vi "LoadProjectSettings.vi"(10 "SeqPath":string, 11 "Sequence Context In":refnum<k7>) -> (0 "error out":errorcluster, 2 "ProjectSettings":T1, 3 "Report Text":string)   [LabVIEW 2018]
uses:
  <vilib>/Utility/config.llb/Read Key (String).vi
  <vilib>/Utility/config.llb/Read Key (U32).vi
  <vilib>/Utility/config.llb/NI_LVConfig.lvlib
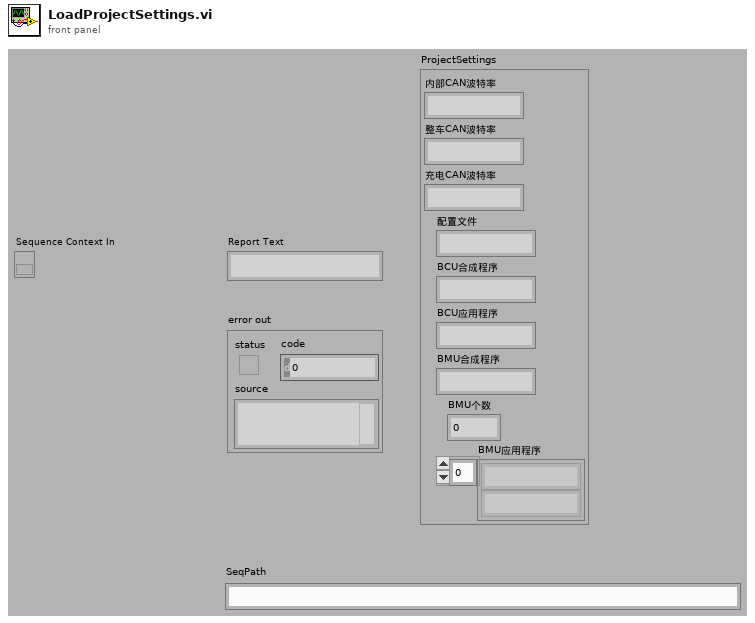
[diagram p1: front panel]
types:
  T1 = cluster{"内部CAN波特率":string, "整车CAN波特率":string, "充电CAN波特率":string, "配置文件":string, "BCU合成程序":string, "BCU应用程序":string, "BMU合成程序":string, "BMU个数":u32, "BMU应用程序":string[]}
  T2 = typedef "NI_LVConfig.lvlib/Config Data RefNum.ctl" = refnum<k1>
  T3 = cluster{"value":string, "value":string, "value":string, string, string, string, string, "value":u32, string[]}
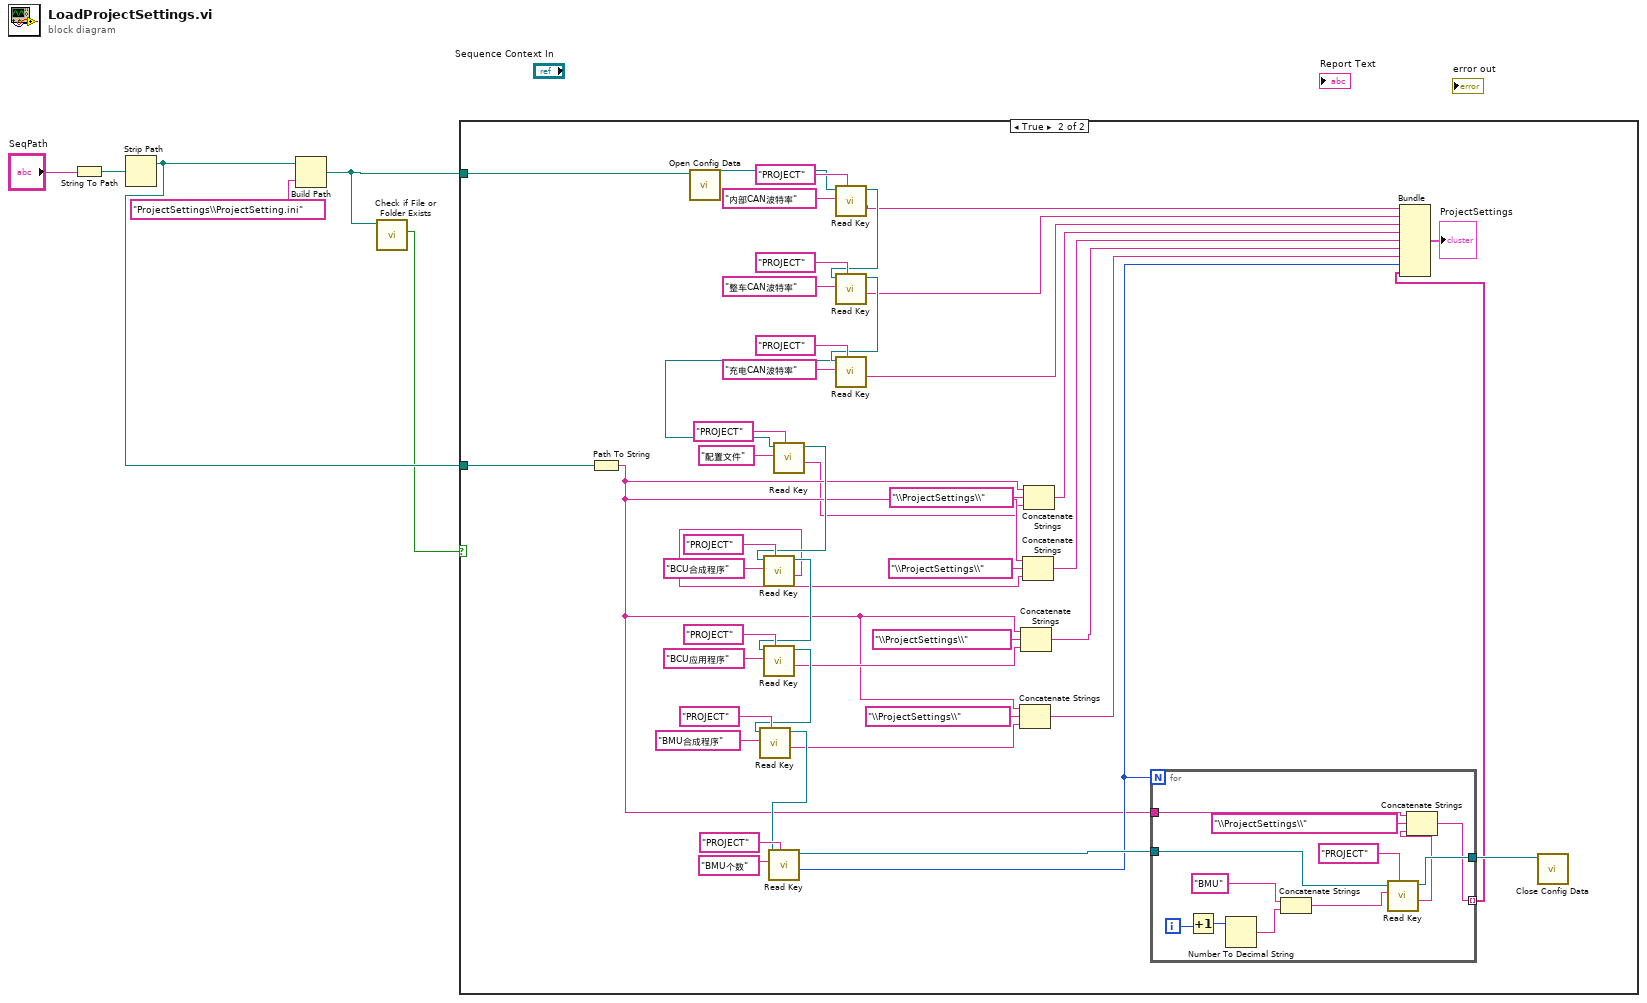
[diagram p0: block diagram]
diagram:
  n1 = String To Path(string="SeqPath") -> (path=w5:path)
  n2 = Strip Path(path=w5) -> (stripped path=w3:path)  [unwired: 1 out]
  n3 = Build Path(base path=w3, name or relative path="ProjectSettings\\ProjectSetting.ini") -> (appended path=w2:path)
  n4 = call <vilib>:"Check if File or Folder Exists.vi"("path"=w2) -> ("file or folder exists?"=w1:bool)  [unwired: 8 in, 2 out]
  n5 = case shown="True" w1 {
    tunnel: w3 -> [_ w22]
    tunnel: w2 -> [_ w8]
    frame False {
    }
    frame True {
      n6 = Path To String(path=w22) -> (string=w11:string)
      n7 = call <vilib>:"Open Config Data.vi"("configuration file path"=w8) -> ("refnum"=w34:T2)  [unwired: 8 in, 2 out]
      n8 = call-poly <vilib>:"Read Key.vi"("section"="PROJECT", "key"="内部CAN波特率", "refnum"=w34) -> ("value"=w7:string, "refnum out"=w47:T2)  [unwired: 5 in, 2 out]
      n9 = call-poly <vilib>:"Read Key.vi"("section"="PROJECT", "key"="整车CAN波特率", "refnum"=w47) -> ("value"=w31:string, "refnum out"=w44:T2)  [unwired: 5 in, 2 out]
      n10 = call-poly <vilib>:"Read Key.vi"("section"="PROJECT", "key"="充电CAN波特率", "refnum"=w44) -> ("value"=w30:string, "refnum out"=w41:T2)  [unwired: 5 in, 2 out]
      n11 = call-poly <vilib>:"Read Key.vi"("section"="PROJECT", "key"="配置文件", "refnum"=w41) -> ("value"=w10:string, "refnum out"=w36:T2)  [unwired: 5 in, 2 out]
      n12 = call-poly <vilib>:"Read Key.vi"("section"="PROJECT", "key"="BCU合成程序", "refnum"=w36) -> ("value"=w20:string, "refnum out"=w35:T2)  [unwired: 5 in, 2 out]
      n13 = call-poly <vilib>:"Read Key.vi"("section"="PROJECT", "key"="BCU应用程序", "refnum"=w35) -> ("value"=w17:string, "refnum out"=w27:T2)  [unwired: 5 in, 2 out]
      n14 = call-poly <vilib>:"Read Key.vi"("section"="PROJECT", "key"="BMU合成程序", "refnum"=w27) -> ("value"=w14:string, "refnum out"=w26:T2)  [unwired: 5 in, 2 out]
      n15 = call-poly <vilib>:"Read Key.vi"("section"="PROJECT", "key"="BMU个数", "refnum"=w26) -> ("value"=w25:u32, "refnum out"=w33:T2)  [unwired: 5 in, 2 out]
      n16 = Concatenate Strings(w11, "\\ProjectSettings\\" ("string"), w14) -> (w13:string)
      n17 = Concatenate Strings(w11, "\\ProjectSettings\\" ("string"), w17) -> (w16:string)
      n18 = Concatenate Strings(w11, "\\ProjectSettings\\" ("string"), w20) -> (w19:string)
      n19 = Concatenate Strings(w11, "\\ProjectSettings\\" ("string"), w10) -> (w9:string)
      n20 = for {
        N: w25 -> [_]
        tunnel: w33 -> [w59]
        tunnel: [w54] -> w24 mode=indexing
        tunnel: [w58] -> w32
        tunnel: w11 -> [w56]
        i -> [w65]
        n21 = Increment(x=w65) -> (x+1=w64:i32)
        n22 = Number To Decimal String(number=w64) -> (decimal integer string=w62:string)  [unwired: 1 in]
        n23 = Concatenate Strings("BMU" ("key"), w62) -> (w60:string)
        n24 = call-poly <vilib>:"Read Key.vi"("section"="PROJECT", "key"=w60, "refnum"=w59) -> ("value"=w55:string, "refnum out"=w58:T2)  [unwired: 5 in, 2 out]
        n25 = Concatenate Strings(w56, "\\ProjectSettings\\" ("string"), w55) -> (w54:string)
      }
      n26 = Bundle("value"=w7, "value"=w31, "value"=w30, w9, w19, w16, w13, "value"=w25, w24) -> (→"ProjectSettings":T3)  [unwired: 1 in]
      n27 = call <vilib>:"Close Config Data.vi"("refnum"=w32) -> ()  [unwired: 9 in, 2 out]
    }
  }
